vi "Rename Variable.vi"(6 "Variable Type":enum16{"Project", "Execution"}(ring), 8 "error in (no error)":errorcluster, 9 "New Name":string, 10 "Current Name":string, 11 "Project in":refnum<class "Project.lvclass">) -> (0 "error out":errorcluster, 1 "Name":string, 2 "Successful":bool, 3 "Project out":refnum<class "Project.lvclass">)   [LabVIEW 2015, in "Project.lvclass"]
uses:
  Project.lvclass
  <vilib>/regexp/Match Regular Expression.xnode
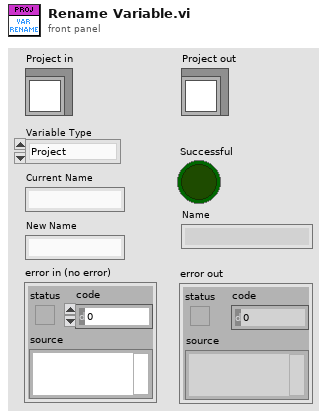
[diagram p1: front panel]
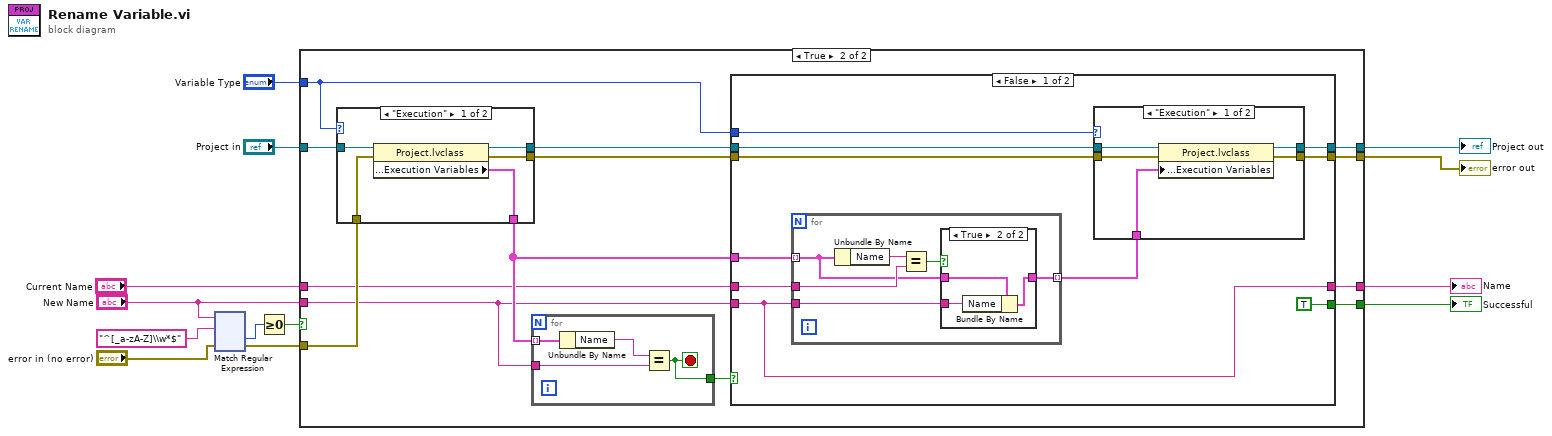
[diagram p0: block diagram]
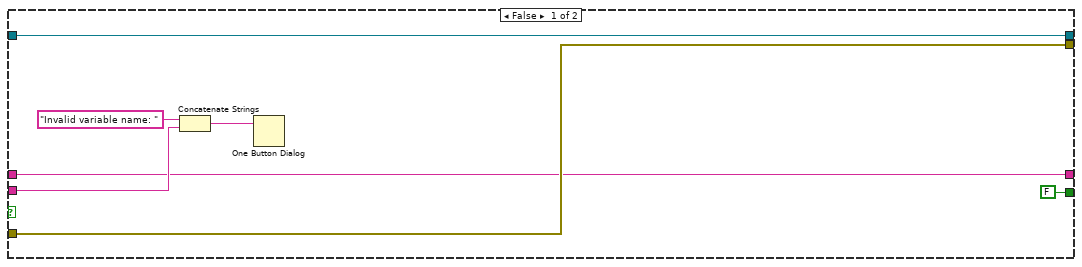
[diagram p2: hidden frame]
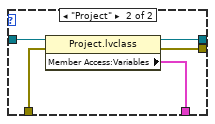
[diagram p3: hidden frame]
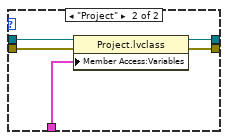
[diagram p4: hidden frame]
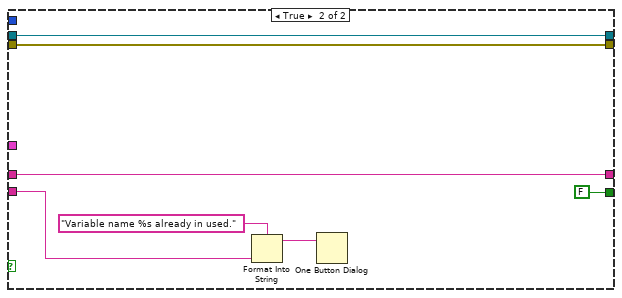
[diagram p6: hidden frame]
diagram:
  n1 = xnode "Match Regular Expression"("input string"="New Name", "regular expression"="^[_a-zA-Z]\\w*$", "error in"="error in (no error)") -> ("offset past match"=w12:i32, "error out"=w7:errorcluster)  [unwired: 3 in, 3 out]
  n2 = Greater Or Equal To 0?(x=w12) -> (x >= 0?=w11:bool)
  n3 = case shown="True" w11 {
    tunnel: "New Name" -> [w19 w29]
    tunnel: "Project in" -> [w17 w33]
    tunnel: w7 -> [w16 w32]
    tunnel: [w17 w26] -> w6
    tunnel: [w16 w25] -> w5
    tunnel: "Variable Type" -> [_ w24]
    tunnel: [FALSE w23] -> w3
    tunnel: "Current Name" -> [w14 w22]
    tunnel: [w14 w21] -> w1
    frame False {
      n4 = Concatenate Strings("Invalid variable name: " ("message"), w19) -> (w18:string)
      n5 = One Button Dialog(message=w18) -> ()  [unwired: 1 in, 1 out]
    }
    frame True {
      n6 = case shown="\"Execution\"" w24 {
        tunnel: w33 -> [w38 w43]
        tunnel: w32 -> [w37 w42]
        tunnel: [w36 w41] -> w30
        tunnel: [w35 w40] -> w28
        tunnel: [w34 w39] -> w27
        frame "Execution" {
          n7 = property class="Project.lvclass"(reference=w38, error in=w37) -> (reference out=w35:refnum<class "Project.lvclass">, error out=w34:errorcluster, "Member Access:Execution Variables"=w36:cluster{"Name":string, "Value":variant}[])
        }
        frame "Project" {
          n8 = property class="Project.lvclass"(reference=w43, error in=w42) -> (reference out=w40:refnum<class "Project.lvclass">, error out=w39:errorcluster, "Member Access:Variables"=w41:cluster{"Name":string, "Value":variant}[])
        }
      }
      n9 = for {
        tunnel: w30 -> [w47] mode=indexing
        tunnel: w29 -> [w45]
        tunnel: [w44] -> w31
        stop <- w44 stop-if-true
        n10 = Unbundle By Name(w47) -> ("Name"=w46:string)
        n11 = Equal?(x=w46, y=w45) -> (x = y?=w44:bool)
      }
      n12 = case shown="False" w31 {
        tunnel: w30 -> [w57 _]
        tunnel: w29 -> [w48 w83]
        tunnel: w22 -> [w56 w78]
        tunnel: w28 -> [w55 w81]
        tunnel: w27 -> [w53 w80]
        tunnel: [w52 w81] -> w26
        tunnel: [w51 w80] -> w25
        tunnel: w24 -> [w50 _]
        tunnel: [TRUE FALSE] -> w23
        tunnel: [w48 w78] -> w21
        frame False {
          n13 = for {
            tunnel: w57 -> [w71] mode=indexing
            tunnel: w56 -> [w72]
            tunnel: w48 -> [w69]
            tunnel: [w68] -> w54 mode=indexing
            n14 = Unbundle By Name(w71) -> ("Name"=w73:string)
            n15 = Equal?(x=w73, y=w72) -> (x = y?=w70:bool)
            n16 = case shown="True" w70 {
              tunnel: w71 -> [w74 w77]
              tunnel: w69 -> [_ w76]
              tunnel: [w74 w75] -> w68
              frame False {
              }
              frame True {
                n17 = Bundle By Name(cluster=w77, "Name"=w76) -> (w75:cluster{"Name":string, "Value":variant})
              }
            }
          }
          n18 = case shown="\"Execution\"" w50 {
            tunnel: w55 -> [w62 w67]
            tunnel: w54 -> [w61 w66]
            tunnel: w53 -> [w60 w65]
            tunnel: [w59 w64] -> w52
            tunnel: [w58 w63] -> w51
            frame "Execution" {
              n19 = property class="Project.lvclass"(reference=w62, error in=w60, "Member Access:Execution Variables"=w61) -> (reference out=w59:refnum<class "Project.lvclass">, error out=w58:errorcluster)
            }
            frame "Project" {
              n20 = property class="Project.lvclass"(reference=w67, error in=w65, "Member Access:Variables"=w66) -> (reference out=w64:refnum<class "Project.lvclass">, error out=w63:errorcluster)
            }
          }
        }
        frame True {
          n21 = Format Into String(format string="Variable name %s already in used." ("message"), w83) -> (resulting string=w82:string)  [unwired: 2 in, 1 out]
          n22 = One Button Dialog(message=w82) -> ()  [unwired: 1 in, 1 out]
        }
      }
    }
  }
  "error out" <- w5
  "Project out" <- w6
  "Successful" <- w3
  "Name" <- w1
